vi "libssh2_knownhost_readline.vi"(8 "error in (no error)":errorcluster, 9 "type (OpenSSH)":T1, 10 "line":string, 11 "known hosts collection":T2) -> (0 "error out":errorcluster)   [LabVIEW 2013, in "libssh2.lvlib"]
doc: "Read a string as if it was a line from a known host file."
uses:
  libssh2.lvlib
  Known Host Collection Refnum.ctl
  Known Host File Type.ctl
  Not A Known Host Collection.vi
  <vilib>/Utility/error.llb/Error Cluster From Error Code.vi
  Global Settings.vi
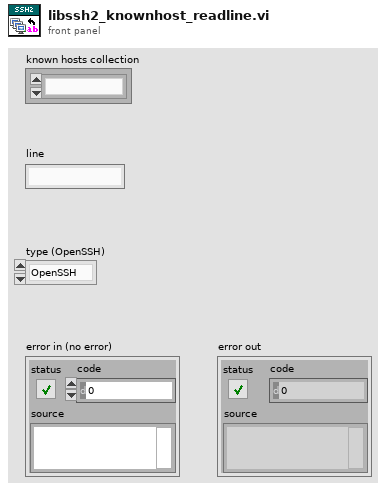
[diagram p1: front panel]
types:
  T1 = typedef "libssh2.lvlib/Known Host File Type.ctl" = enum16{"OpenSSH"}
  T2 = typedef "libssh2.lvlib/Known Host Collection Refnum.ctl" = refnum<k1>
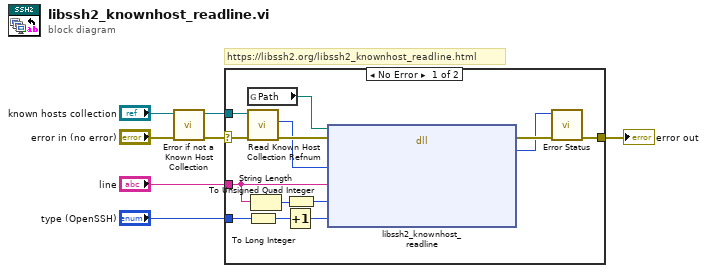
[diagram p0: block diagram]
diagram:
  # "https://libssh2.org/libssh2_knownhost_readline.html"
  n1 = call "Error if not a Known Host Collection.vi"("error in (no error)"="error in (no error)", "known host collection"="known hosts collection") -> ("error out"=w3:errorcluster, "known host collection out"=w1:T2)  [unwired: 8 in]
  n2 = case shown="No Error" w3 {
    selector: w3 -> [w20 w22]
    tunnel: [w19 w22] -> w7
    tunnel: "line" -> [w10 _]
    tunnel: "type (OpenSSH)" -> [w21 _]
    tunnel: w1 -> [w18 _]
    frame No Error {
      n3 = global read "Global Settings.vi" "Path"() -> (w14:path)
      n4 = call "Read Known Host Collection Refnum.vi"("error in (no error)"=w20, "known hosts collection"=w18) -> ("error out"=w16:errorcluster, "LIBSSH2_KNOWNHOSTS*"=w15:u64)  [unwired: 8 in]
      n5 = To Long Integer(number=w21) -> (32bit integer=w12:i32)
      n6 = String Length(string=w10) -> (length=w9:i32)
      n7 = Increment(x=w12) -> (x+1=w11:i32)
      n8 = To Unsigned Quad Integer(1:w9) -> (0:w8:u64)
      n9 = dll-call lib="?" fn="libssh2_knownhost_readline"(path in=w14, error in=w16, "hosts"=w15, "line"=w10, "len"=w8, "type"=w11) -> (error out=w17:errorcluster, "return value"=w13:i32)  [unwired: 5 in, 1 out]
      n10 = call "Error Status.vi"("error in (no error)"=w17, "return value"=w13) -> ("error out"=w19:errorcluster)  [unwired: 8 in, 1 out]
    }
    frame Error {
    }
  }
  "error out" <- w7
